vi "draw_overlay_in_physical_coordinates.vi"(0 "Image in":refnum<class "Image.lvclass">, 1 "x offset":dbl[unit], 2 "y offset":dbl[unit], 3 "overlay group":string, 5 "x coordinates":dbl[unit][](array[numeric]), 7 "y coordinates":dbl[unit][](array[numeric]), 11 "error in (no error)":errorcluster, 12 "colour":u32(colorbox)=16711680, 13 "origin":T1, 14 "clear previous overlay of this group?":bool=TRUE) -> (4 "Image out":refnum<class "Image.lvclass">, 15 "error out":errorcluster)   [LabVIEW 2010, in "Image.lvclass"]
uses:
  Image.lvclass
  origin_type_enum.ctl
  ErrorController/ErrorController/class_data.vi
  ErrorController/ErrorController/ErrorController.lvclass
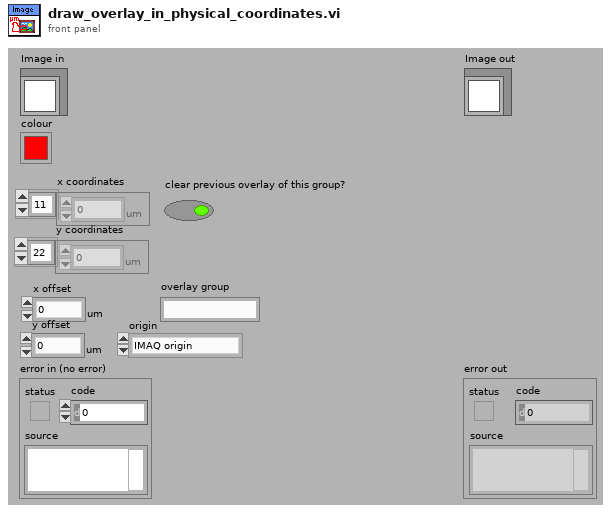
[diagram p1: front panel]
types:
  T1 = typedef "origin_type_enum.ctl" = enum16{"IMAQ origin", "middle of image"}
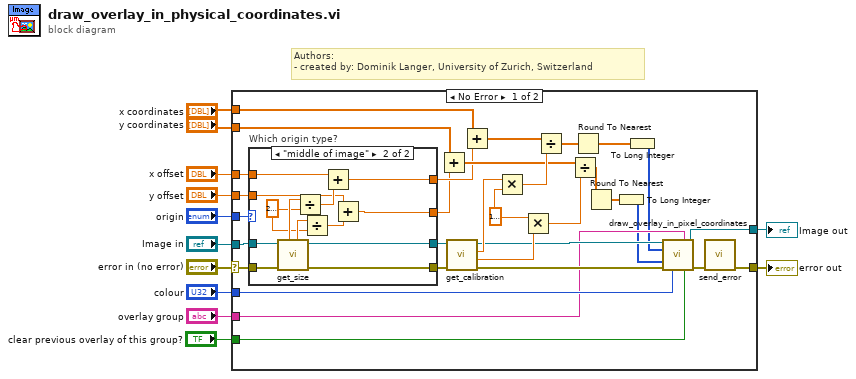
[diagram p0: block diagram]
diagram:
  # "Authors: \n- created by: Dominik Langer, University of Zurich, Switzerland"
  n1 = case shown="No Error" "error in (no error)" {
    selector: "error in (no error)" -> [w31 w63]
    tunnel: [w13 w63] -> w11
    tunnel: [w37 w62] -> w9
    tunnel: "Image in" -> [w30 w62]
    tunnel: "y coordinates" -> [w33 _]
    tunnel: "x coordinates" -> [w35 _]
    tunnel: "colour" -> [w36 _]
    tunnel: "x offset" -> [w25 _]
    tunnel: "y offset" -> [w26 _]
    tunnel: "origin" -> [w27 _]
    tunnel: "overlay group" -> [w22 _]
    tunnel: "clear previous overlay of this group?" -> [w21 _]
    frame No Error {
      w40 = dbl[unit] 1e-06 ("y")
      n2 = case "Which origin type?" shown="\"middle of image\"" w27 {
        tunnel: w31 -> [w47 w61]
        tunnel: w30 -> [w48 w60]
        tunnel: [w47 w59] -> w29
        tunnel: [w48 w58] -> w28
        tunnel: w26 -> [w45 w51]
        tunnel: w25 -> [w46 w52]
        tunnel: [w45 w50] -> w23
        tunnel: [w46 w49] -> w24
        frame "IMAQ origin", Default {
        }
        frame "middle of image" {
          w55 = dbl[unit] 2000000.0 ("y")
          n3 = call-dynamic "get_size.vi"("error in (no error)"=w61, "Image in"=w60) -> ("error out"=w59:errorcluster, "Image out"=w58:refnum<class "Image.lvclass">, "physical size y"=w56:dbl, "physical size x"=w57:dbl)  [unwired: 2 in, 4 out]
          n4 = Divide(x=w57, y=w55) -> (x/y=w54:dbl[unit])
          n5 = Divide(x=w56, y=w55) -> (x/y=w53:dbl[unit])
          n6 = Add(x=w52, y=w54) -> (x+y=w49:dbl[unit])
          n7 = Add(x=w51, y=w53) -> (x+y=w50:dbl[unit])
        }
      }
      n8 = Add(x=w33, y=w23) -> (x+y=w32:dbl[unit][])
      n9 = call "get_calibration.vi"("error in (no error)"=w29, "Image.lvclass in"=w28) -> ("error out"=w44:errorcluster, "y"=w41:dbl, "x"=w43:dbl, "Image.lvclass out"=w38:refnum<class "Image.lvclass">)  [unwired: 4 in, 2 out]
      n10 = Add(x=w35, y=w24) -> (x+y=w34:dbl[unit][])
      n11 = Multiply(x=w43, y=w40) -> (x*y=w42:dbl[unit])
      n12 = Multiply(x=w40, y=w41) -> (x*y=w39:dbl[unit])
      n13 = Divide(x=w34, y=w42) -> (x/y=w20:dbl[])
      n14 = Divide(x=w32, y=w39) -> (x/y=w19:dbl[])
      n15 = Round To Nearest(number=w20) -> (nearest integer value=w18:dbl[])
      n16 = Round To Nearest(number=w19) -> (nearest integer value=w17:dbl[])
      n17 = To Long Integer(number=w17) -> (32bit integer=w16:i32[])
      n18 = To Long Integer(number=w18) -> (32bit integer=w15:i32[])
      n19 = call "draw_overlay_in_pixel_coordinates.vi"("Image in"=w38, "overlay group"=w22, "x coordinates"=w15, "y coordinates"=w16, "error in (no error)"=w44, "colour"=w36, "clear previous overlay of this group? (T)"=w21) -> ("Image out"=w37:refnum<class "Image.lvclass">, "error out"=w14:errorcluster)  [unwired: 7 in]
      n20 = call "send_error.vi"("error in (no error)"=w14) -> ("error out"=w13:errorcluster)  [unwired: 10 in]
    }
    frame Error {
    }
  }
  "error out" <- w11
  "Image out" <- w9
